vi "Pre-Build VI - Run Unit Tests.vi"(8 "error in (no error)":errorcluster, 11 "Fail on #todo items":bool) -> (0 "error out":errorcluster, 1 "VIs without test coverage":string[](array[string]), 2 "error type":enum16{"fatal", "non-fatal", "warning"}(ring), 3 "num tests":i32, 4 "VIs not loadable":string[](array[string]), 5 "VIs Failed":string[](array[string]), 6 "VIs with #todo bookmarks":string[](array[string]))   [LabVIEW 2020]
uses:
  <vilib>/Utility/miscctls.llb/LVBookmarkInfoTypeDef.ctl
  <vilib>/addons/_JKI Toolkits/Caraya/run-tests/Run Test (Scalar Path).vi
  <vilib>/addons/_JKI Toolkits/Caraya/Caraya.lvlib
panel:
  out "VIs with #todo's":map{path, T1}(c390)
  out "VIs Succeeded":string[](array[string])
  in  "type specifier VI Refnum (for type only)":refnum<vi>
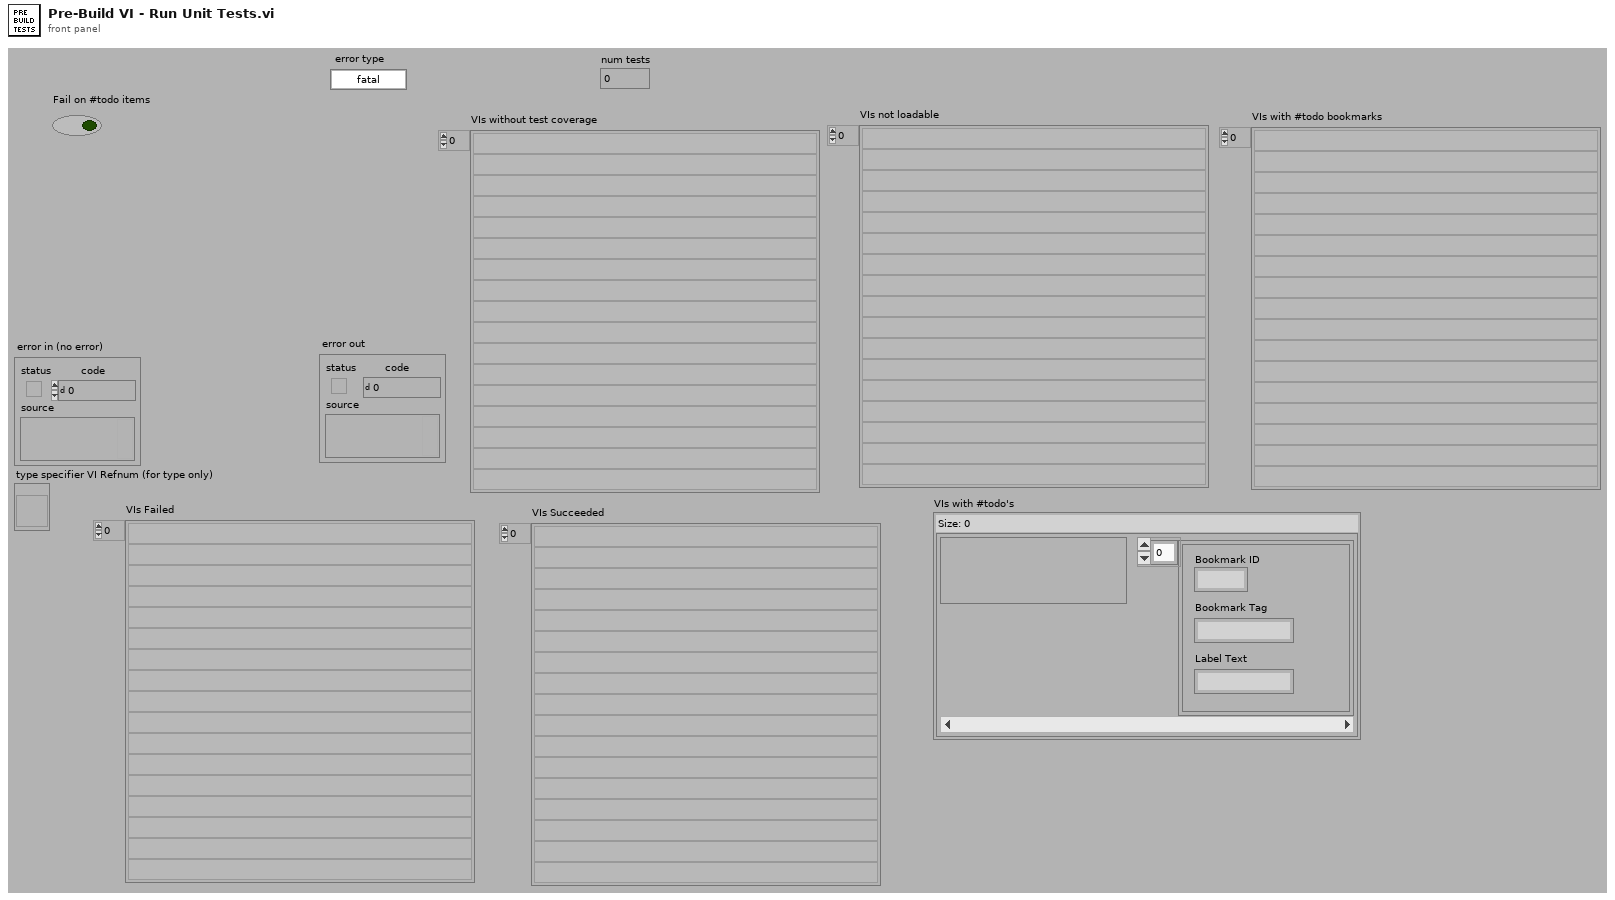
[diagram p1: front panel]
types:
  T1 = typedef "LVBookmarkInfoTypeDef.ctl" = cluster{"Bookmark ID":u32, "Bookmark Tag":string, "Label Text":string}[]
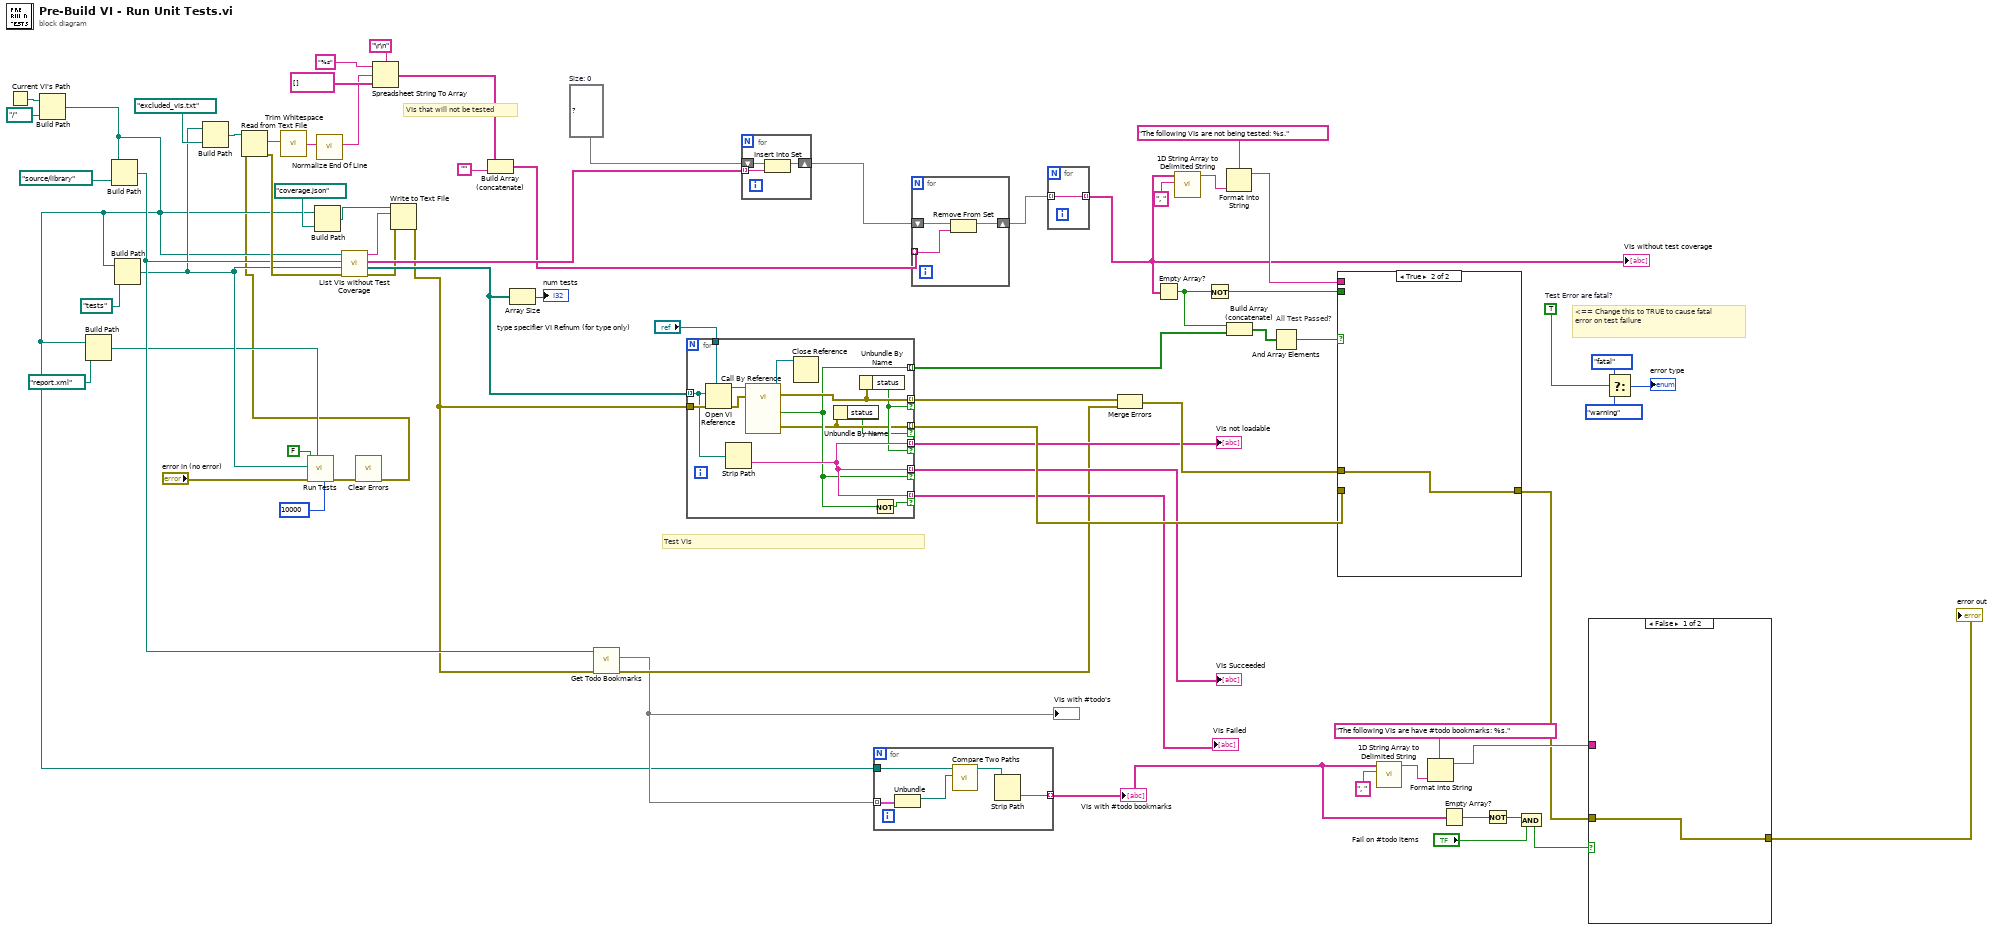
[diagram p0: block diagram]
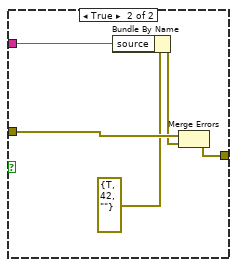
[diagram p2: hidden frame]
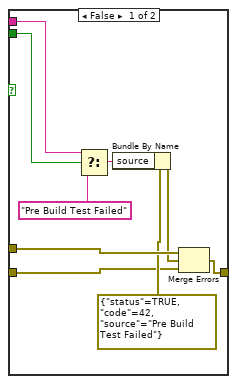
[diagram p3: hidden frame]
diagram:
  w45 = set{string} {}  # Size: 0
  w64 = TRUE  # Test Error are fatal?
  # "VIs that will not be tested"
  # "<== Change this to TRUE to cause fatal error on test failure"
  # "All Test Passed?"
  # "Test VIs"
  n1 = Current VI's Path() -> (path=w51:path)
  n2 = Build Path(base path=w51, name or relative path=path "../..") -> (appended path=w2:path)
  n3 = Build Path(base path=w2, name or relative path=path "report.xml" ("Relative path (.)")) -> (appended path=w12:path)
  n4 = Build Path(base path=w2, name or relative path=path "source/library" ("Relative path (.)")) -> (appended path=w29:path)
  n5 = Build Path(base path=w2, name or relative path=path "tests" ("Relative path (.)")) -> (appended path=w15:path)
  n6 = Build Path(base path=w15, name or relative path=path "excluded_vis.txt" ("Relative path (.)")) -> (appended path=w46:path)
  n7 = call-poly <vilib>:"Run Tests.vi"("timeout (2000 ms)"=10000, "Report Path"=w12, "error in"="error in (no error)", "Test Path"=w15, "Interactive (T)"=FALSE) -> ("error out"=w9:errorcluster)  [unwired: 5 in, 1 out]
  n8 = Build Path(base path=w2, name or relative path=path "coverage.json" ("Relative path (.)")) -> (appended path=w6:path)
  n9 = call <vilib>:"Clear Errors.vi"("error in (no error)"=w9) -> ("error out"=w1:errorcluster)  [unwired: 5 in, 1 out]
  n10 = Read from Text File(file (use dialog)=w46, error in=w1) -> (text=w33:string, error out=w32:errorcluster)  [unwired: 2 in, 2 out]
  n11 = call <vilib>:"Trim Whitespace.vi"("string"=w33) -> ("trimmed string"=w35:string)  [unwired: 1 in]
  n12 = call <vilib>:"Normalize End Of Line.vi"("string in"=w35) -> ("string out"=w34:string)  [unwired: 7 in]
  n13 = call "List VIs without Test Coverage.vi"("error in (no error)"=w32, "Tests Root"=w15, "Source Root"=w29, "Project Root"=w2) -> ("error out"=w4:errorcluster, "Test VIs"=w31:path[], "VIs without test coverage"=w44:string[], "coverage.json"=w5:string)  [unwired: 4 in]
  n14 = Spreadsheet String To Array(delimiter (Tab)="\r\n", format string="%s", spreadsheet string=w34, array type (2D Dbl)=string[] [] ("appended array")) -> (array=w36:string[])
  n15 = Write to Text File(file (use dialog)=w6, text=w5, error in=w4) -> (error out=w3:errorcluster)  [unwired: 1 in, 2 out]
  n16 = Build Array (concatenate)(w36, "") -> (w42:string[])
  n17 = Array Size(array=w31) -> (size(s)=→"num tests":i32)
  n18 = call "Get Todo Bookmarks.vi"("error in (no error)"=w3, "Directory to Search"=w29) -> ("error out"=w28:errorcluster, "todo bookmarks"=w19:map{path, T1})  [unwired: 8 in]
  "VIs with #todo's" <- w19
  n19 = for {
    tunnel: w31 -> [w78] mode=indexing
    tunnel: "type specifier VI Refnum (for type only)" -> [w84]
    tunnel: [w76] -> w55 mode=indexing
    tunnel: [w73] -> w59 mode=indexing if=w72
    tunnel: w3 -> [w80]
    tunnel: [w79] -> w56 mode=indexing if=w74
    tunnel: [w77] -> w54 mode=indexing if=w74
    tunnel: [w77] -> w53 mode=indexing if=w76
    tunnel: [w77] -> w52 mode=indexing if=w75
    n20 = Open VI Reference(type specifier VI Refnum (for type only)=w84, vi path=w78, error in (no error)=w80) -> (vi reference=w83:refnum<vi>, error out=w82:errorcluster)  [unwired: 3 in]
    n21 = Strip Path(path=w78) -> (name=w77:string)  [unwired: 1 out]
    n22 = call-by-ref "?"(reference=w83, error in=w82) -> (reference out=w81:refnum<vi>, error out=w79:errorcluster, 0:"error out"=w73:errorcluster, "pass"=w76:bool)  [unwired: 10 in]
    n23 = Close Reference(reference=w81) -> ()  [unwired: 1 in, 1 out]
    n24 = Unbundle By Name(w73) -> ("status"=w72:bool)
    n25 = Unbundle By Name(w79) -> ("status"=w74:bool)
    n26 = Not(x=w76) -> (.not. x?=w75:bool)
  }
  "VIs not loadable" <- w54
  "VIs Succeeded" <- w53
  "VIs Failed" <- w52
  n27 = for {
    tunnel: w44 -> [w87] mode=indexing
    shift-right: [w85] -> w43
    shift-left: w45 -> [w86]
    n28 = Insert Into Set(10:w87, 11:w86) -> (3:w85:set{string})  [unwired: 1 out]
  }
  n29 = for {
    tunnel: w19 -> [w92] mode=indexing
    tunnel: w2 -> [w90]
    tunnel: [w88] -> w22 mode=indexing
    n30 = Unbundle(w92) -> ("key type"=w91:path)  [unwired: 1 out]
    n31 = call <vilib>:"Compare Two Paths.vi"("Path 2"=w91, "Path 1"=w90) -> ("Relative Path from 1 to 2"=w89:path)  [unwired: 6 in, 3 out]
    n32 = Strip Path(path=w89) -> (name=w88:string)  [unwired: 1 out]
  }
  "VIs with #todo bookmarks" <- w22
  n33 = for {
    shift-right: [w93] -> w41
    shift-left: w43 -> [w95]
    tunnel: w42 -> [w94] mode=indexing
    n34 = Remove From Set(10:w94, 11:w95) -> (3:w93:set{string})  [unwired: 1 out]
  }
  n35 = for {
    tunnel: [w96] -> w40 mode=indexing
    tunnel: w41 -> [w96] mode=indexing
  }
  "VIs without test coverage" <- w40
  n36 = Merge Errors(w56, w28) -> (w57:errorcluster)
  n37 = Empty Array?(array=w40) -> (empty?=w66:bool)
  n38 = call <vilib>:"1D String Array to Delimited String.vi"("delimiter"=", " ("delimiter (Tab)"), "string array"=w40) -> ("delimited string"=w69:string)  [unwired: 9 in]
  n39 = Not(x=w66) -> (.not. x?=w65:bool)
  n40 = Format Into String(format string="The following VIs are not being tested: %s.", w69) -> (resulting string=w67:string)  [unwired: 2 in, 1 out]
  n41 = Build Array (concatenate)(w66, w55) -> (w27:bool[])
  n42 = And Array Elements(Boolean array=w27) -> (logical AND=w71:bool)
  n43 = case shown="True" w71 {
    tunnel: w57 -> [w105 w106]
    tunnel: [w104 w106] -> w20
    tunnel: w65 -> [w103 _]
    tunnel: w67 -> [w102 _]
    tunnel: w59 -> [w97 _]
    frame False {
      n44 = Select(t=w102, s=w103, f="Pre Build Test Failed" ("source")) -> (s? t:f=w100:string)
      n45 = Bundle By Name(cluster=errorcluster {"status"=TRUE, "code"=42, "source"="Pre Build Test Failed"} ("error out"), "source"=w100) -> (w99:errorcluster)
      n46 = Merge Errors(w105, w99, w97) -> (w104:errorcluster)
    }
    frame True {
    }
  }
  n47 = call <vilib>:"1D String Array to Delimited String.vi"("delimiter"=", " ("delimiter (Tab)"), "string array"=w22) -> ("delimited string"=w25:string)  [unwired: 9 in]
  n48 = Format Into String(format string="The following VIs are have #todo bookmarks: %s.", w25) -> (resulting string=w23:string)  [unwired: 2 in, 1 out]
  n49 = Empty Array?(array=w22) -> (empty?=w21:bool)
  n50 = Not(x=w21) -> (.not. x?=w18:bool)
  n51 = And(x=w18, y="Fail on #todo items") -> (x .and. y?=w17:bool)
  n52 = case shown="False" w17 {
    tunnel: w20 -> [w107 w112]
    tunnel: [w107 w108] -> w8
    tunnel: w23 -> [_ w109]
    frame False {
    }
    frame True {
      n53 = Bundle By Name(cluster=errorcluster {"status"=TRUE, "code"=42, "source"=""} ("error out"), "source"=w109) -> (w111:errorcluster)
      n54 = Merge Errors(w112, w111) -> (w108:errorcluster)
    }
  }
  "error out" <- w8
  n55 = Select(t=enum16{"fatal", "non-fatal", "warning"}."fatal" ("error type"), s=w64, f=enum16{"fatal", "non-fatal", "warning"}."warning" ("error type")) -> (s? t:f=→"error type":enum16{"fatal", "non-fatal", "warning"})
